vi "JPEG string to LV Image.vi"(0 "JPEG String":string, 11 "error in":errorcluster) -> (6 "LV Image":T1, 15 "error out":errorcluster)   [LabVIEW 2020]
doc: "Uses .NET functions to convert a GIF file to a PNG file"
uses:
  <vilib>/picture/picture.llb/imagedata.ctl
  System.Drawing
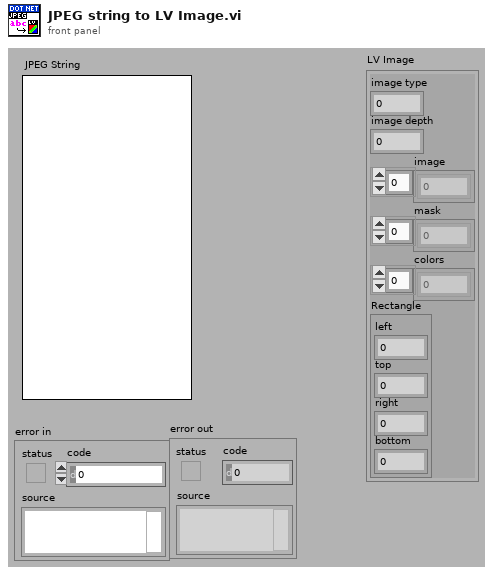
[diagram p1: front panel]
types:
  T1 = typedef "imagedata.ctl" = cluster{"image type":i32, "image depth":i32, "image":u8[], "mask":u8[], "colors":u32[], "Rectangle":cluster{"left":i16, "top":i16, "right":i16, "bottom":i16}}
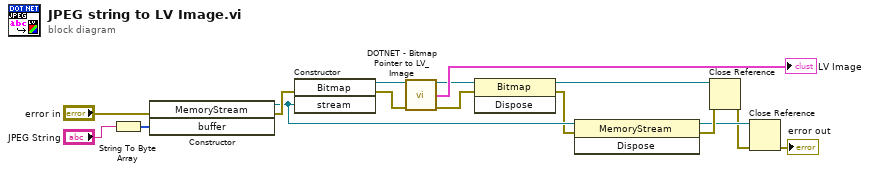
[diagram p0: block diagram]
diagram:
  n1 = String To Byte Array(string="JPEG String") -> (unsigned byte array=w15:u8[])
  n2 = constructor class="MemoryStream"(error in="error in", "buffer"=w15) -> (reference out=w9:refnum<k24>, error out=w13:errorcluster)  [unwired: 2 in, 2 out]
  n3 = constructor class="Bitmap"(error in=w13, "stream"=w9) -> (reference out=w12:refnum<k24>, error out=w11:errorcluster)  [unwired: 2 in, 2 out]
  n4 = call "DOTNET - Bitmap Pointer to LV_Image.vi"("Bitmap"=w12, "error in (no error)"=w11) -> ("Bitmap dup"=w8:refnum<k24>, "LV_Image"=→"LV Image":T1, "error out"=w7:errorcluster)  [unwired: 10 in, 1 out]
  n5 = invoke class="Bitmap" method="Dispose"(reference=w8, error in=w7) -> (reference out=w5:refnum<k24>, error out=w6:errorcluster)  [unwired: 1 in, 1 out]
  n6 = invoke class="MemoryStream" method="Dispose"(reference=w9, error in=w6) -> (reference out=w3:refnum<k24>, error out=w4:errorcluster)  [unwired: 1 in, 1 out]
  n7 = Close Reference(reference=w5, error in (no error)=w4) -> (error out=w2:errorcluster)
  n8 = Close Reference(reference=w3, error in (no error)=w2) -> (error out=→"error out":errorcluster)
